vi "Matrix Rotation.vi"(8 "Error In":errorcluster caption="Entrée d'erreur", 9 "Rot Mat":T2=[[0.0, -1.0], [1.0, 0.0]], 10 "Pivot":T2=[[1.5], [1.5]], 11 "Coordinates":T1[](array[typedef])) -> (0 "Error Out":errorcluster caption="Sortie d'erreur", 3 "Rotated Coordinates":T1[](array[typedef]))   [LabVIEW 2017]
uses:
  Controls/Coordinates.ctl
  <vilib>/Analysis/Matrix/Datatypes/RealMatrix.ctl
  <vilib>/Analysis/Matrix/Numeric/Subtract/Subtract - RM,RM.vi
  <vilib>/Analysis/Matrix/Numeric/Multiply/Multiply - RM,RM.vi
  <vilib>/Analysis/Matrix/Numeric/Add/Add - RM,RM.vi
  <vilib>/Analysis/Matrix/NI_Matrix.lvlib
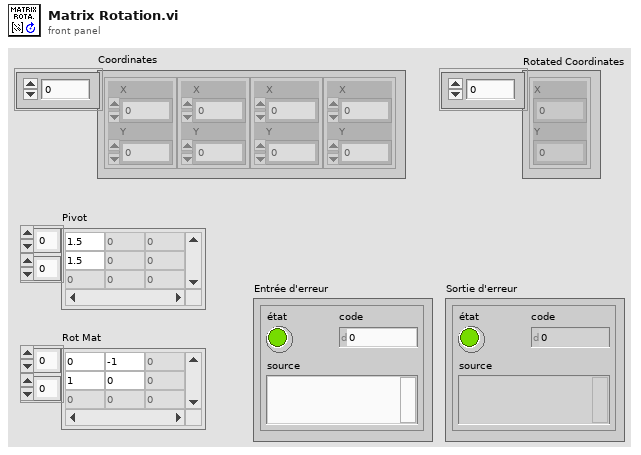
[diagram p1: front panel]
types:
  T1 = typedef "Coordinates.ctl" = cluster{"X":i32, "Y":i32}
  T2 = typedef "NI_Matrix.lvlib/RealMatrix.ctl" = dbl[][]
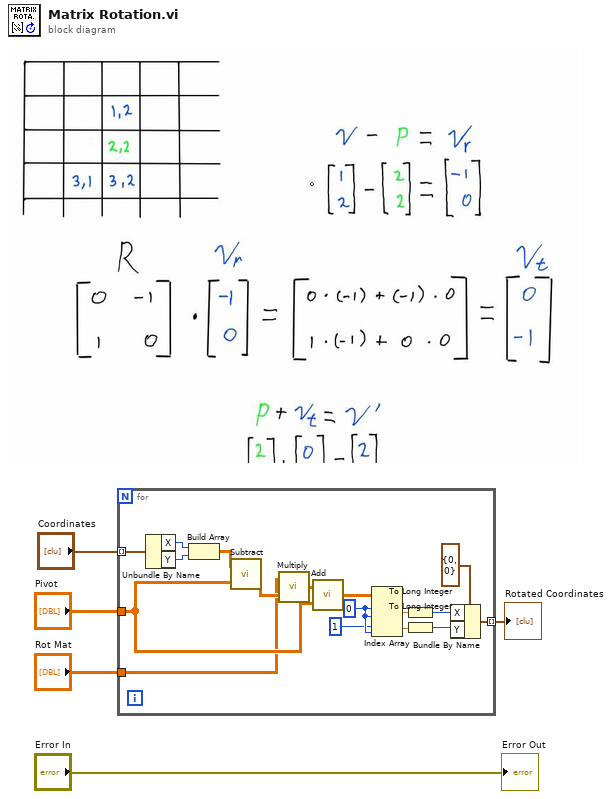
[diagram p0: block diagram]
diagram:
  n1 = for {
    tunnel: "Coordinates" -> [w22] mode=indexing
    tunnel: "Pivot" -> [w16]
    tunnel: "Rot Mat" -> [w15]
    tunnel: [w6] -> w2 mode=indexing
    w13 = 0 ("indice (ligne)")
    n2 = Unbundle By Name(w22) -> ("X"=w21:i32, "Y"=w20:i32)
    n3 = Build Array(w21, w20) -> (w19:T2)
    n4 = call-poly <vilib>:"Subtract.vi"("Real Matrix B"=w16, "Real Matrix A"=w19) -> ("A - B"=w17:T2)
    n5 = call-poly <vilib>:"Multiply.vi"("Real Matrix B"=w17, "Real Matrix A"=w15) -> ("A * B"=w18:T2)
    n6 = call-poly <vilib>:"Add.vi"("Real Matrix B"=w16, "Real Matrix A"=w18) -> ("A + B"=w14:T2)
    n7 = Index Array(array=w14, index (row) #1=w13, index (col) #1=w13, index (row) #2=1 ("indice (ligne)"), index (col) #2=w13) -> (element #1=w11:dbl, element #2=w10:dbl)
    n8 = To Long Integer(number=w11) -> (32bit integer=w9:i32)
    n9 = To Long Integer(number=w10) -> (32bit integer=w7:i32)
    n10 = Bundle By Name(cluster=T1 {"X"=0, "Y"=0} ("Coordinates"), "X"=w9, "Y"=w7) -> (w6:T1)
  }
  "Rotated Coordinates" <- w2
  "Error Out" <- "Error In"
